vi "From Serial Form.vi"(6 "Serial Version":T1, 10 "Deserializer in":refnum<class "Deserializer.lvclass">, 11 "Iterator in":refnum<class "Iterator.lvclass">) -> (0 "error out":errorcluster, 2 "Deserializer out":refnum<class "Deserializer.lvclass">, 3 "Iterator out":refnum<class "Iterator.lvclass">)   [LabVIEW 2015, in "Iterator.lvclass"]
uses:
  Iterator.lvclass
  <vilib>/NI/AQ Character Lineator/Deserializer/Deserializer.lvclass
  <vilib>/NI/AQ Character Lineator/Serialization Common/Serial Version.ctl
  <vilib>/NI/AQ Character Lineator/Serializable/Serializable.lvclass
  <vilib>/NI/AQ Character Lineator/Serialization Common/Serialization Common.lvlib
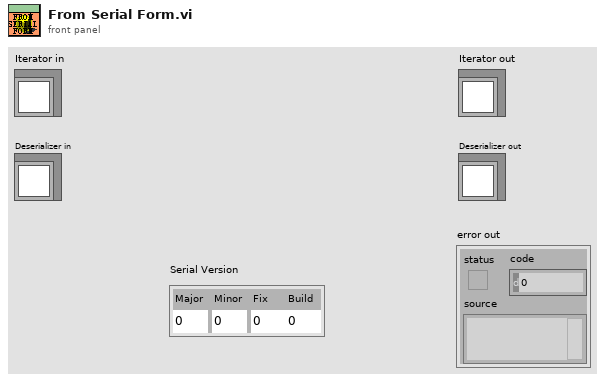
[diagram p1: front panel]
types:
  T1 = typedef "Serialization Common.lvlib/Serial Version.ctl" = cluster{"Major":u16, "Minor":u16, "Fix":u16, "Build":u16}
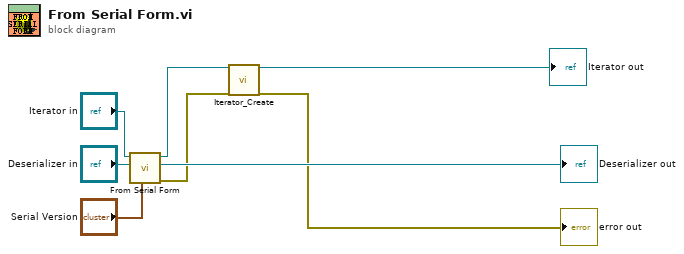
[diagram p0: block diagram]
diagram:
  n1 = call-parent "From Serial Form.vi"("Serial Version"="Serial Version", "Deserializer in"="Deserializer in", "Serializable in"="Iterator in") -> ("error out"=w3:errorcluster, "Deserializer out"=→"Deserializer out":refnum<class "Deserializer.lvclass">, "Serializable out"=w4:refnum<class "Iterator.lvclass">)  [unwired: 6 in]
  n2 = call "Iterator_Create.vi"("reference in"=w4, "error in (no error)"=w3) -> ("reference out"=→"Iterator out":refnum<class "Iterator.lvclass">, "error out"=→"error out":errorcluster)  [unwired: 16 in]
